vi "dataUserOut.vi"(8 "error in (no error)":errorcluster) -> (0 "error out":errorcluster, 3 "Data":string[][](array[string]))   [LabVIEW 2014]
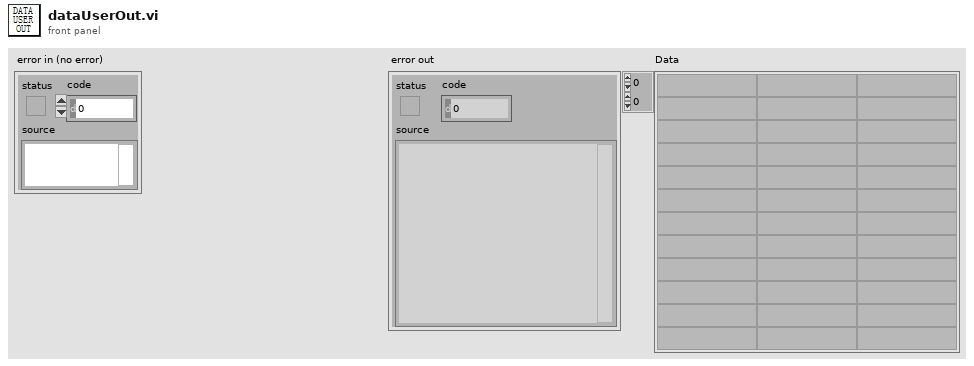
[diagram p1: front panel]
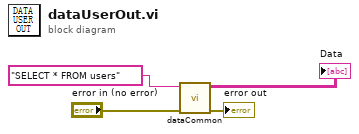
[diagram p0: block diagram]
diagram:
  n1 = call "dataCommon.vi"("error in (no error)"="error in (no error)", "Command Text"="SELECT * FROM users" ("SQL query")) -> ("error out"=→"error out":errorcluster, "Data"=→"Data":string[][])  [unwired: 8 in]
